vi "Simple UDP - Sender.vi"() -> ()   [LabVIEW 2016]
doc: "The UDP protocol differs from TCP in that there is no error-checking with the packets of information that are sent, and thus no guarantee whatsoever that an intended recipient will actually receive a given piece of data.\n\nUDP does offer the ability to \"broadcast\" data across a network--simply specify an IP Address of all ones (255.255.255.255) to attempt to broadcast information network-wide. Keep in mind that routers and other network hardware will generally refuse to forward the broadcast beyond certain points, so the extent of the broadcast will in practice be limited."
panel:
  in  "address to write to":string="10.0.95.67"
  in  "remote port":u16=61557
  in  "Values to Write":dbl[](array[numeric])=[1.0, 2.0]
  in  "Stop":bool
  # "Overview: Demonstrates the use of the UDP functions to send data over a UDP connection.\nInstructions:\n1. Run the VI.\n2. Open Simple UDP - Receiver.vi and follow the instructions on its front panel.\n3. Click Stop to stop the VI."
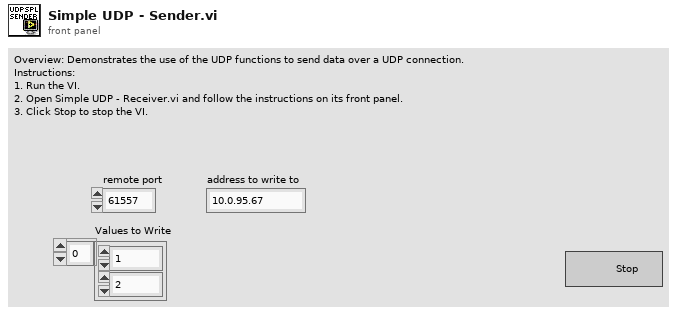
[diagram p1: front panel]
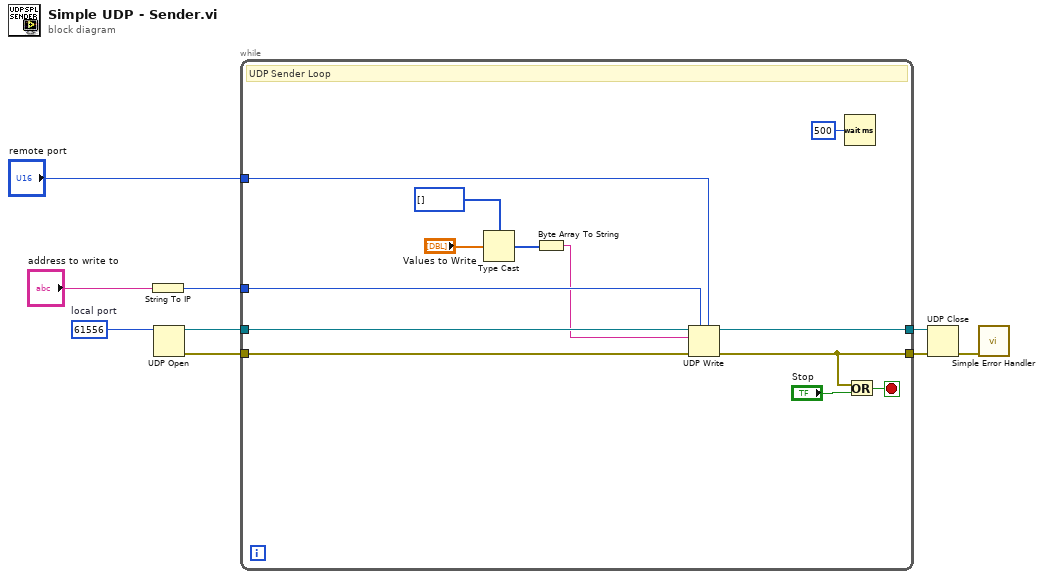
[diagram p0: block diagram]
diagram:
  w2 = u16 61556  # local port
  n1 = String To IP(1:"address to write to") -> (0:w5:u32)
  n2 = UDP Open(11:w2) -> (port=w4:refnum<k16>, 0:w3:errorcluster)  [unwired: 4 in, 1 out]
  n3 = while {
    tunnel: [w17] -> w8
    tunnel: w4 -> [w22]
    tunnel: w3 -> [w21]
    tunnel: [w18] -> w9
    tunnel: w5 -> [w16]
    tunnel: "remote port" -> [w15]
    stop <- w20 stop-if-true
    # "UDP Sender Loop"
    n4 = Type Cast(type=u8[] [], x="Values to Write") -> (*(type *) &x=w11:u8[])
    n5 = Byte Array To String(unsigned byte array=w11) -> (string=w10:string)
    n6 = UDP Write(address=w16, port or service name=w15, connection ID=w22, data in=w10, 8:w21) -> (error out=w17:errorcluster, 3:w18:refnum<k16>)  [unwired: 1 in]
    n7 = Wait (ms)(milliseconds to wait=u32 500) -> ()  [unwired: 1 out]
    n8 = Or(x=w17, y="Stop") -> (x .or. y?=w20:bool)
  }
  n9 = UDP Close(connection ID=w9, 8:w8) -> (error out=w6:errorcluster)  [unwired: 1 out]
  n10 = call <vilib>:"Simple Error Handler.vi"("error in (no error)"=w6) -> ()  [unwired: 4 in, 5 out]
